vi "S2C_InitGlobals.vi"(8 "Error In":errorcluster) -> (0 "Error Out":errorcluster)   [LabVIEW 2015]
doc: "Initializes front panel globals."
uses:
  Core/Command/S2C_CMD_Globals.vi
  AccessDB/S2C_Access_Globals.vi
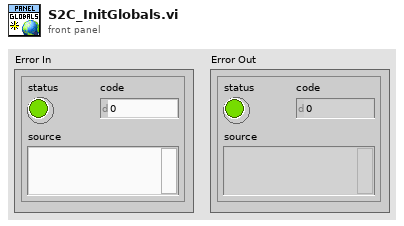
[diagram p1: front panel]
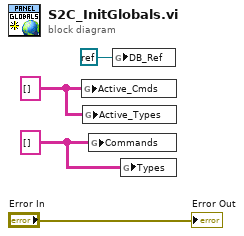
[diagram p0: block diagram]
diagram:
  w3 = string[][][][] [] ("Commands")
  w4 = string[][][] [] ("Active_Cmds")
  n1 = global write "S2C_CMD_Globals.vi" "Active_Cmds"(w4) -> ()
  n2 = global write "S2C_CMD_Globals.vi" "Active_Types"(w4) -> ()
  n3 = global write "S2C_CMD_Globals.vi" "Commands"(w3) -> ()
  n4 = global write "S2C_Access_Globals.vi" "DB_Ref"(refnum<k0> refnum) -> ()
  n5 = global write "S2C_CMD_Globals.vi" "Types"(w3) -> ()
  "Error Out" <- "Error In"
